vi "SubtractU8Baseline.vi"(10 "Baseline U8":u8, 11 "New samples in":u64) -> (3 "New samples out":u64)   [LabVIEW 2012]
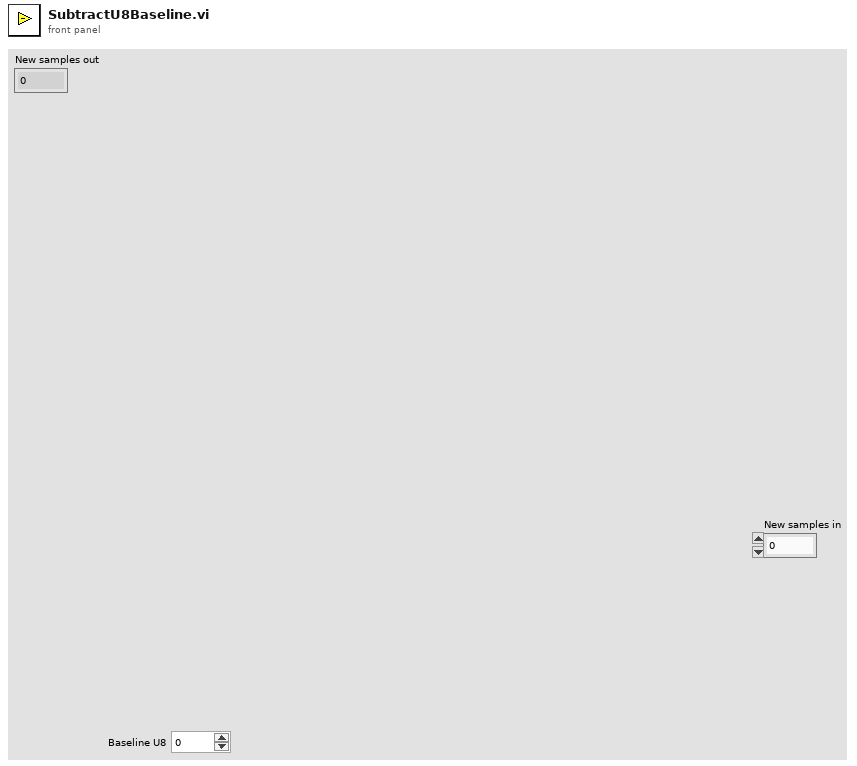
[diagram p1: front panel]
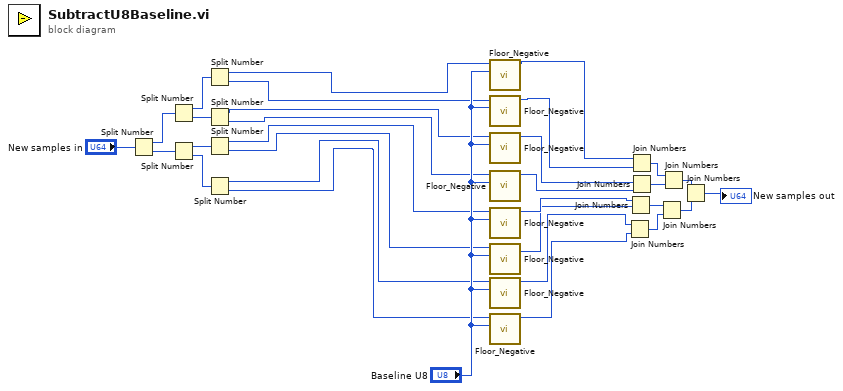
[diagram p0: block diagram]
diagram:
  n1 = Split Number(x="New samples in") -> (hi(x)=w15:u32, lo(x)=w14:u32)
  n2 = Split Number(x=w15) -> (hi(x)=w13:u16, lo(x)=w12:u16)
  n3 = Split Number(x=w14) -> (hi(x)=w11:u16, lo(x)=w10:u16)
  n4 = Split Number(x=w13) -> (hi(x)=w9:u8, lo(x)=w8:u8)
  n5 = Split Number(x=w12) -> (hi(x)=w7:u8, lo(x)=w6:u8)
  n6 = Split Number(x=w11) -> (hi(x)=w5:u8, lo(x)=w4:u8)
  n7 = Split Number(x=w10) -> (hi(x)=w3:u8, lo(x)=w2:u8)
  n8 = call "Floor_Negative.vi"("Baseline U8"="Baseline U8", "Input Value"=w9) -> ("Output Value"=w24:u8)  [unwired: 9 in]
  n9 = call "Floor_Negative.vi"("Baseline U8"="Baseline U8", "Input Value"=w8) -> ("Output Value"=w23:u8)  [unwired: 9 in]
  n10 = call "Floor_Negative.vi"("Baseline U8"="Baseline U8", "Input Value"=w7) -> ("Output Value"=w22:u8)  [unwired: 9 in]
  n11 = call "Floor_Negative.vi"("Baseline U8"="Baseline U8", "Input Value"=w6) -> ("Output Value"=w21:u8)  [unwired: 9 in]
  n12 = call "Floor_Negative.vi"("Baseline U8"="Baseline U8", "Input Value"=w5) -> ("Output Value"=w20:u8)  [unwired: 9 in]
  n13 = call "Floor_Negative.vi"("Baseline U8"="Baseline U8", "Input Value"=w4) -> ("Output Value"=w19:u8)  [unwired: 9 in]
  n14 = call "Floor_Negative.vi"("Baseline U8"="Baseline U8", "Input Value"=w3) -> ("Output Value"=w18:u8)  [unwired: 9 in]
  n15 = call "Floor_Negative.vi"("Baseline U8"="Baseline U8", "Input Value"=w2) -> ("Output Value"=w17:u8)  [unwired: 9 in]
  n16 = Join Numbers(hi=w18, lo=w17) -> ((hi.lo)=w27:u16)
  n17 = Join Numbers(hi=w20, lo=w19) -> ((hi.lo)=w28:u16)
  n18 = Join Numbers(hi=w24, lo=w23) -> ((hi.lo)=w30:u16)
  n19 = Join Numbers(hi=w22, lo=w21) -> ((hi.lo)=w29:u16)
  n20 = Join Numbers(hi=w28, lo=w27) -> ((hi.lo)=w25:u32)
  n21 = Join Numbers(hi=w30, lo=w29) -> ((hi.lo)=w26:u32)
  n22 = Join Numbers(hi=w26, lo=w25) -> ((hi.lo)=→"New samples out":u64)
